vi "S2C_PCIe7841_Proc_PortWrite.vi"(8 "Error In":errorcluster, 11 "Data":string) -> (0 "Error Out":errorcluster)   [LabVIEW 2015]
uses:
  S2C_PCIe7841_Proc_Globals.vi
  <vilib>/Utility/error.llb/Error Cluster From Error Code.vi
  <vilib>/rvi/errors/niLvFpgaAdjustHostInterfaceError.vi
  <vilib>/rvi/interface/nirviMethod/nirviMethod.xnode
  <vilib>/FPGAPlugInAG/Dynamic/niLvFpga_WriteFifo_Dynamic.vi
  <vilib>/rvi/errors/niLvFpgaMergeErrorWithErrorCode.vi
panel:
  out "Conn":u8
  out "Data":u16 format="%016b"
  out "Size":bool
  out "State":bool
  out "Port":bool[](array[boolean])
  out "Bits":bool[](array[boolean])
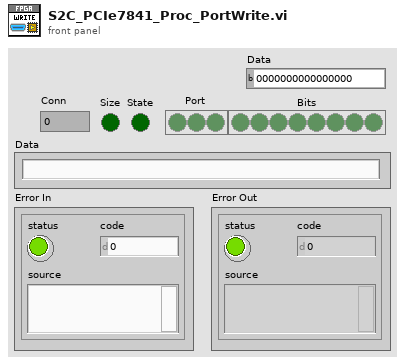
[diagram p1: front panel]
types:
  T1 = cluster{"Connector":u8, "Port":u8, "Data":string}
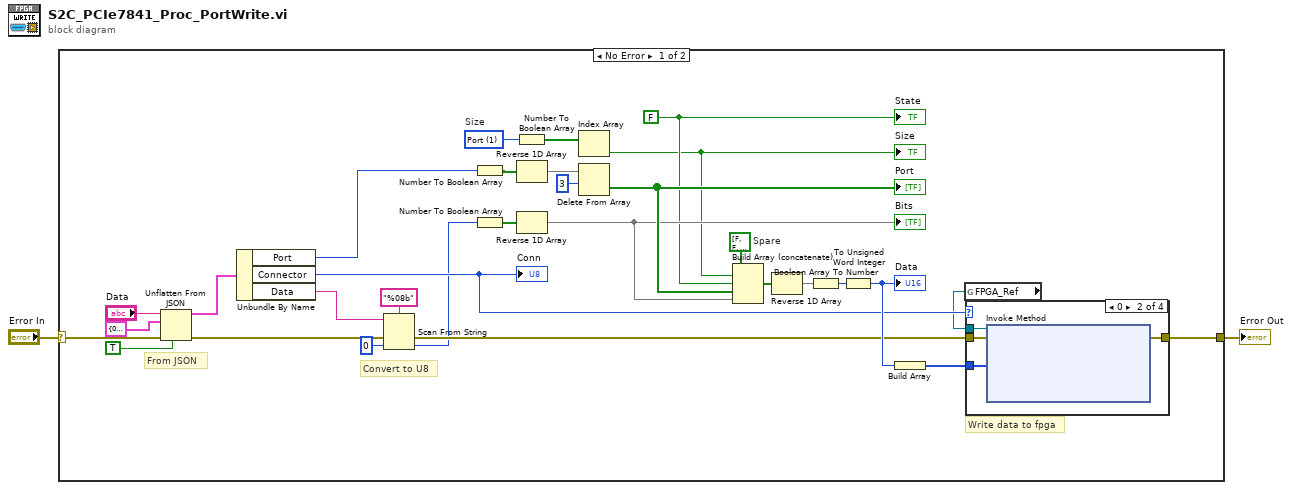
[diagram p0: block diagram]
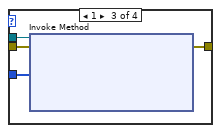
[diagram p3: hidden frame]
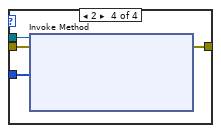
[diagram p4: hidden frame]
diagram:
  n1 = case shown="No Error" "Error In" {
    selector: "Error In" -> [w33 w47]
    tunnel: [w16 w47] -> w1
    frame No Error {
      w5 = FALSE ("element")
      w9 = u8 1 items=["Bit", "Port"]  # Size
      w25 = bool[] [FALSE, FALSE, FALSE, FALSE]  # Spare
      # "Write data to fpga"
      # "From JSON"
      # "Convert to U8"
      n2 = Unflatten From JSON(JSON string="Data", type and defaults=T1 {"Connector"=0, "Port"=0, "Data"=""}, default null elements? (F)=TRUE, error in (no error)=w33) -> (value=w30:T1, error out=w14:errorcluster)  [unwired: 3 in]
      n3 = Unbundle By Name(w30) -> ("Port"=w7:u8, "Connector"=w8:u8, "Data"=w13:string)
      "Conn" <- w8
      n4 = Scan From String(format string="%08b", input string=w13, error in=w14, default 1=u8 0) -> (error out=w11:errorcluster, output 1=w6:u8)  [unwired: 1 in, 2 out]
      n5 = Number To Boolean Array(number=w7) -> (Boolean array=w27:bool[])
      n6 = Number To Boolean Array(number=w6) -> (Boolean array=w28:bool[])
      n7 = Number To Boolean Array(number=w9) -> (Boolean array=w10:bool[])
      n8 = Reverse 1D Array(array=w27) -> (reversed array=w26:bool[])
      n9 = Reverse 1D Array(array=w28) -> (reversed array=w19:bool[])
      "Bits" <- w19
      n10 = Index Array(array=w10) -> (element=w4:bool)  [unwired: 1 in]
      "Size" <- w4
      n11 = Delete From Array(array=w26, length=3) -> (deleted portion=w20:bool[])  [unwired: 1 in, 1 out]
      "Port" <- w20
      n12 = Build Array (concatenate)(w25, w4, w5, w20, w19) -> (w24:bool[])
      n13 = Reverse 1D Array(array=w24) -> (reversed array=w22:bool[])
      n14 = Boolean Array To Number(Boolean array=w22) -> (number=w23:u32)
      n15 = To Unsigned Word Integer(number=w23) -> (unsigned 16bit integer=w18:u16)
      "Data" <- w18
      n16 = Build Array(w18) -> (w17:u16[])
      n17 = global read "S2C_PCIe7841_Proc_Globals.vi" "FPGA_Ref"() -> (w3:refnum<k20>)
      n18 = case shown="0" w8 {
        tunnel: w11 -> [w34 w38 w42 w46]
        tunnel: w17 -> [_ w37 w41 w45]
        tunnel: [w34 w36 w40 w44] -> w16
        tunnel: w3 -> [_ w35 w39 w43]
        frame 4, Default {
        }
        frame 0 {
          n19 = xnode "Invoke Method"("FPGA VI Reference In"=w35, "error in"=w38, "Data"=w37) -> ("error out"=w36:errorcluster)  [unwired: 1 in, 2 out]
        }
        frame 1 {
          n20 = xnode "Invoke Method"("FPGA VI Reference In"=w39, "error in"=w42, "Data"=w41) -> ("error out"=w40:errorcluster)  [unwired: 1 in, 2 out]
        }
        frame 2 {
          n21 = xnode "Invoke Method"("FPGA VI Reference In"=w43, "error in"=w46, "Data"=w45) -> ("error out"=w44:errorcluster)  [unwired: 1 in, 2 out]
        }
      }
      "State" <- w5
    }
    frame Error {
    }
  }
  "Error Out" <- w1
